vi "SetMatlabParametersFromTypeAndName.vi"(6 "Label.Text":string, 9 "Value":variant, 10 "MatlabType":u16, 11 "ExperimentID":string) -> ()   [LabVIEW 2017]
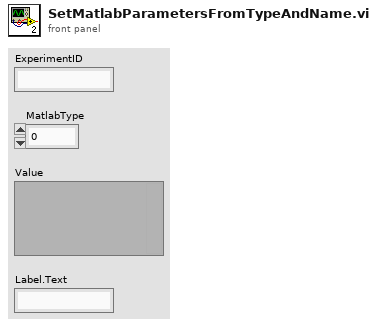
[diagram p1: front panel]
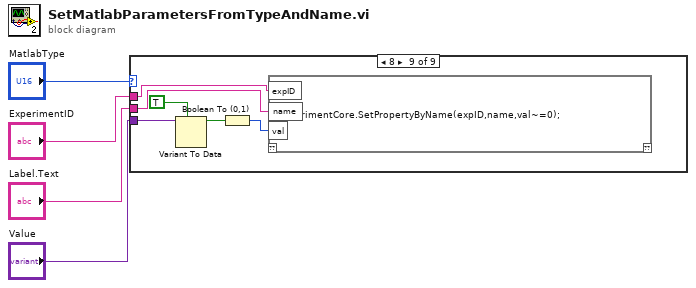
[diagram p0: block diagram]
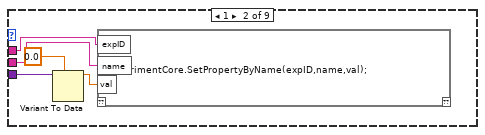
[diagram p3: hidden frame]
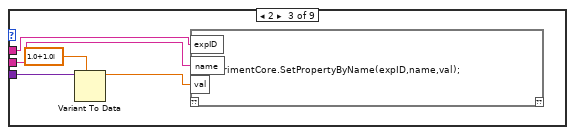
[diagram p4: hidden frame]
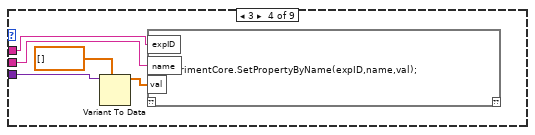
[diagram p5: hidden frame]
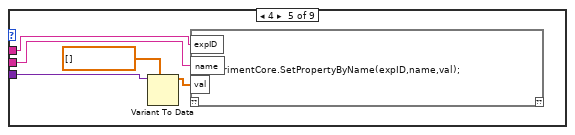
[diagram p6: hidden frame]
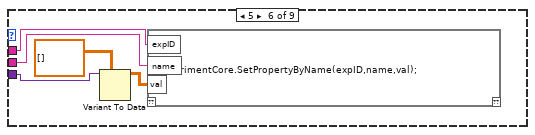
[diagram p7: hidden frame]
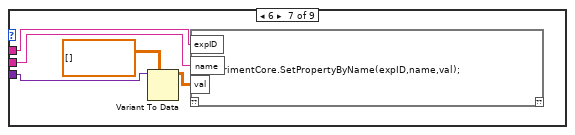
[diagram p8: hidden frame]
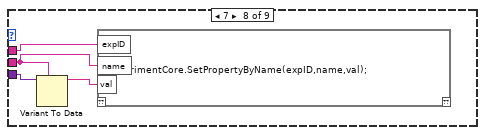
[diagram p9: hidden frame]
diagram:
  n1 = case shown="8" "MatlabType" {
    tunnel: "Value" -> [_ w9 w14 w19 w24 w29 w34 w38 w44]
    tunnel: "Label.Text" -> [_ w8 w13 w18 w23 w28 w33 w36 w42]
    tunnel: "ExperimentID" -> [_ w7 w12 w17 w22 w27 w32 w37 w43]
    frame 0, Default {
    }
    frame 1 {
      n2 = Variant To Data(type=0.0, Variant=w9) -> (data=w5:dbl)  [unwired: 1 in, 1 out]
      n3 = script code="ExperimentCore.SetPropertyByName(expID,name,val);"("expID"=w7, "name"=w8, "val"=w5) -> ()  [unwired: 1 in, 1 out]
    }
    frame 2 {
      n4 = Variant To Data(type=cdb 1.0+1.0i, Variant=w14) -> (data=w11:cdb)  [unwired: 1 in, 1 out]
      n5 = script code="ExperimentCore.SetPropertyByName(expID,name,val);"("expID"=w12, "name"=w13, "val"=w11) -> ()  [unwired: 1 in, 1 out]
    }
    frame 3 {
      n6 = Variant To Data(type=dbl[] [], Variant=w19) -> (data=w16:dbl[])  [unwired: 1 in, 1 out]
      n7 = script code="ExperimentCore.SetPropertyByName(expID,name,val);"("expID"=w17, "name"=w18, "val"=w16) -> ()  [unwired: 1 in, 1 out]
    }
    frame 4 {
      n8 = Variant To Data(type=cdb[] [], Variant=w24) -> (data=w21:cdb[])  [unwired: 1 in, 1 out]
      n9 = script code="ExperimentCore.SetPropertyByName(expID,name,val);"("expID"=w22, "name"=w23, "val"=w21) -> ()  [unwired: 1 in, 1 out]
    }
    frame 5 {
      n10 = Variant To Data(type=dbl[][] [], Variant=w29) -> (data=w25:dbl[][])  [unwired: 1 in, 1 out]
      n11 = script code="ExperimentCore.SetPropertyByName(expID,name,val);"("expID"=w27, "name"=w28, "val"=w25) -> ()  [unwired: 1 in, 1 out]
    }
    frame 6 {
      n12 = Variant To Data(type=cdb[][] [], Variant=w34) -> (data=w31:cdb[][])  [unwired: 1 in, 1 out]
      n13 = script code="ExperimentCore.SetPropertyByName(expID,name,val);"("expID"=w32, "name"=w33, "val"=w31) -> ()  [unwired: 1 in, 1 out]
    }
    frame 7 {
      n14 = Variant To Data(type=w36, Variant=w38) -> (data=w35:string)  [unwired: 1 in, 1 out]
      n15 = script code="ExperimentCore.SetPropertyByName(expID,name,val);"("expID"=w37, "name"=w36, "val"=w35) -> ()  [unwired: 1 in, 1 out]
    }
    frame 8 {
      n16 = Variant To Data(type=TRUE, Variant=w44) -> (data=w40:bool)  [unwired: 1 in, 1 out]
      n17 = Boolean To (0,1)(Boolean=w40) -> (0, 1=w39:i16)
      n18 = script code="ExperimentCore.SetPropertyByName(expID,name,val~=0);"("expID"=w43, "name"=w42, "val"=w39) -> ()  [unwired: 1 in, 1 out]
    }
  }
